vi "StorePAQsample.vi"(8 "error in (no error)":errorcluster, 10 "PAQ IN":T1 {"data" format="%.2f"; "status" format="%08x"}, 11 "HISW in":refnum<class "HISW.lvclass">) -> (0 "error out":errorcluster, 3 "HISW out":refnum<class "HISW.lvclass">)   [LabVIEW 2020, in "Sgraph_lib_V1.lvlib" / "HISW.lvclass"]
doc: "Process one PAQ datagram as received from the HISW DAQ Queue\nThis VI depends on the AVPP postprocessor to determine where and how to save the data using FAMM.\n\nThis routine will store one PAQ sample to the data historian.\nIf the TAG does not exist: then it will be created.\nThe time of calling this routine is utilized as measurement time.\n\n- Medium speed acquisition (around 6 s/min up to 10 s/sec)\n - Continuous acquisition\n - Usual fixed acquisition speed\n - One timestamp per sample of multiple channels\n - All channels sampled simultaneous\n - Usual non-deterministic (not real time)\n - Typical application field: DCS or MES systems"
uses:
  HISW.lvclass
  D:/Labview/Sgraph/Sgraph/source/AVPP/AVPP.lvclass
  controls/typedef_PAQsample.ctl
  controls/typedef_PAQdatagram.ctl
  AVPP/AVPP.lvclass
panel:
  # "Write Continuous Perioc data to Historian"
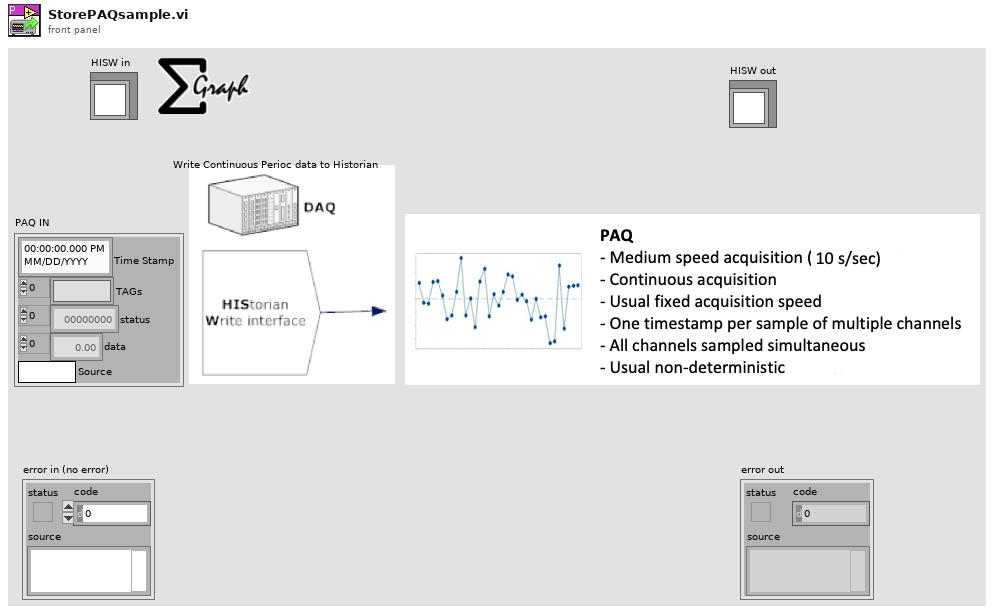
[diagram p1: front panel]
types:
  T1 = typedef "typedef_PAQsample.ctl" = cluster{"Time Stamp":timestamp, "TAGs":string[], "status":u32[], "data":dbl[], "Source":string}
  T2 = typedef "typedef_PAQdatagram.ctl" = cluster{"Time":timestamp, "TAGidx":i32[], "status":u32[], "data":dbl[], "Source":string}
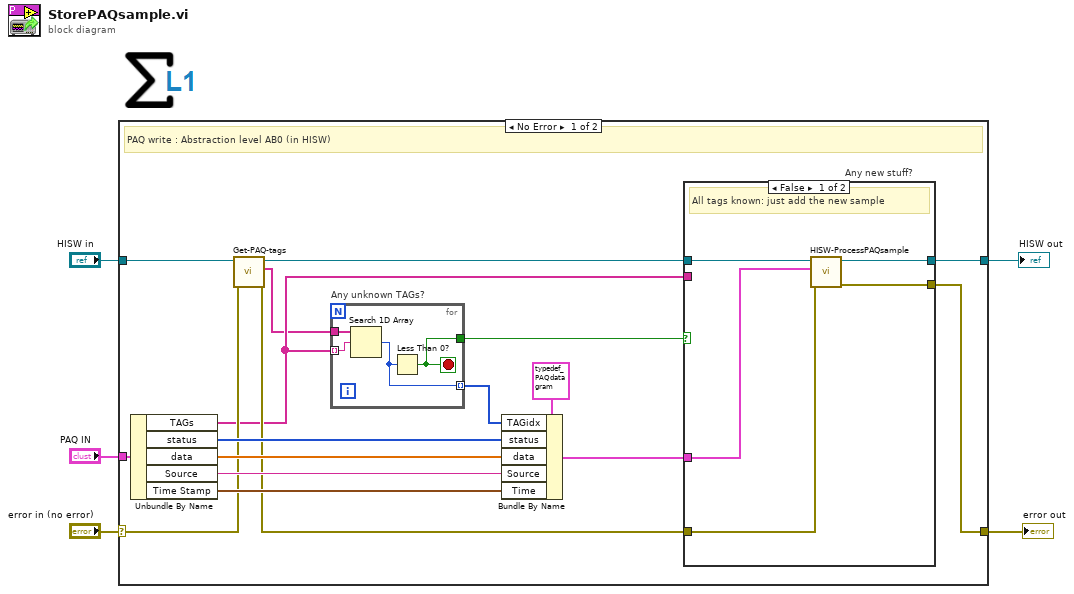
[diagram p0: block diagram]
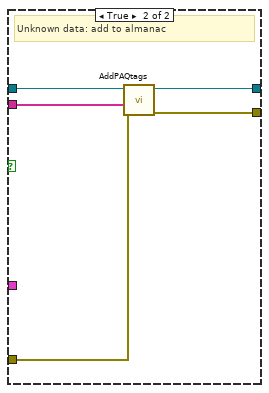
[diagram p2: hidden frame]
diagram:
  n1 = case shown="No Error" "error in (no error)" {
    selector: "error in (no error)" -> [w12 w38]
    tunnel: [w8 w38] -> w4
    tunnel: [w9 w37] -> w1
    tunnel: "HISW in" -> [w13 w37]
    tunnel: "PAQ IN" -> [w22 _]
    frame No Error {
      # "PAQ write : Abstraction level AB0 (in HISW)"
      n2 = Unbundle By Name(w22) -> ("TAGs"=w7:string[], "status"=w19:u32[], "data"=w18:dbl[], "Source"=w17:string, "Time Stamp"=w14:timestamp)
      n3 = call "Get-PAQ-tags.vi"("error in (no error)"=w12, "HISW in"=w13) -> ("error out"=w11:errorcluster, "PAQ_TAGs"=w6:string[], "HISW out"=w10:refnum<class "HISW.lvclass">)  [unwired: 7 in]
      n4 = for "Any unknown TAGs?" {
        tunnel: w6 -> [w36]
        tunnel: w7 -> [w35] mode=indexing
        tunnel: [w34] -> w16
        tunnel: [w33] -> w20 mode=indexing
        stop <- w34 stop-if-true
        n5 = Search 1D Array(1D array=w36, element=w35) -> (index of element=w33:i32)  [unwired: 1 in]
        n6 = Less Than 0?(x=w33) -> (x < 0?=w34:bool)
      }
      n7 = Bundle By Name(cluster=T2 {"Time"=timestamp(0 s since 1904-01-01), "TAGidx"=[], "status"=[], "data"=[], "Source"=""} ("PAQsample"), "TAGidx"=w20, "status"=w19, "data"=w18, "Source"=w17, "Time"=w14) -> (w15:T2)
      n8 = case "Any new stuff?" shown="False" w16 {
        tunnel: w10 -> [w27 w31]
        tunnel: [w26 w30] -> w9
        tunnel: w11 -> [w24 w32]
        tunnel: w7 -> [_ w28]
        tunnel: w15 -> [w23 _]
        tunnel: [w25 w29] -> w8
        frame False {
          # "All tags known: just add the new sample"
          n9 = call "HISW-ProcessPAQsample.vi"("error in (no error)"=w24, "PAQdatagram IN"=w23, "HISW in"=w27) -> ("error out"=w25:errorcluster, "HISW out"=w26:refnum<class "HISW.lvclass">)  [unwired: 7 in]
        }
        frame True {
          # "Unknown data: add to almanac"
          n10 = call "AddPAQtags.vi"("error in (no error)"=w32, "TAGs"=w28, "AVPP in"=w31) -> ("error out"=w29:errorcluster, "AVPP out"=w30:refnum<class "HISW.lvclass">)  [unwired: 7 in]
        }
      }
    }
    frame Error {
    }
  }
  "error out" <- w4
  "HISW out" <- w1
